vi "BuildInstaller.vi"(6 "VersionString":string, 8 "error in":errorcluster, 9 "DestinationDir":path, 10 "BuildSpec":string, 11 "ProjectPath":path=path "C:/Users/pauloneill/SCC/Orion/LabVIEW/Source/App/Orion.lvproj") -> (0 "error out":errorcluster, 3 "Generated files":path[](array[path]))   [LabVIEW 2020, in "CICD.lvlib"]
doc: "Build Windows Installer."
uses:
  CICD.lvlib
  <vilib>/AppBuilder/AB_API_Simple/NI_App_Builder_API.lvlib
  <vilib>/AppBuilder/AB_API_Simple/Build (path).vi
  <vilib>/AppBuilder/AB_API_Simple/Set Build Specification Version (path).vi
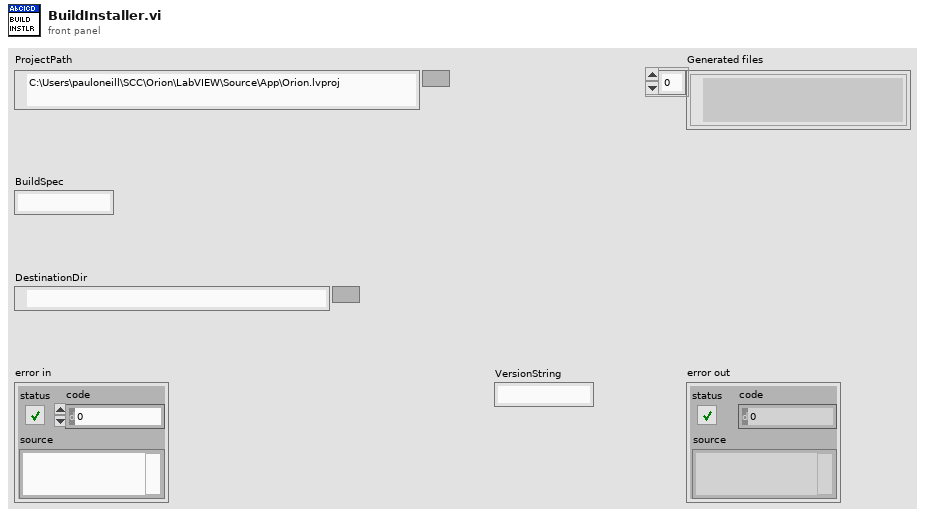
[diagram p1: front panel]
types:
  T1 = typedef "NI_App_Builder_API.lvlib/Build Specification Version.ctl" = cluster{"Major":u16, "Minor":u16, "Fix":u16, "Build":u16}
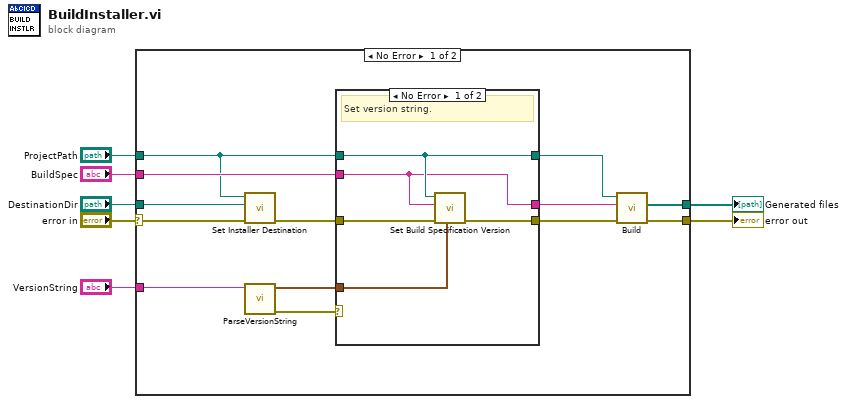
[diagram p0: block diagram]
diagram:
  n1 = case shown="No Error" "error in" {
    selector: "error in" -> [w12 w29]
    tunnel: [w19 w29] -> w7
    tunnel: "ProjectPath" -> [w10 _]
    tunnel: "BuildSpec" -> [w17 _]
    tunnel: "VersionString" -> [w16 _]
    tunnel: [w13 _] -> w3
    tunnel: "DestinationDir" -> [w9 _]
    frame No Error {
      n2 = call "Set Installer Destination.vi"("error in"=w12, "INST_buildLocation"=w9, ".lvproj"=w10) -> ("error out"=w11:errorcluster)  [unwired: 8 in]
      n3 = call "ParseVersionString.vi"("VersionString"=w16) -> ("error out"=w18:errorcluster, "Build spec version"=w8:T1)  [unwired: 9 in]
      n4 = case shown="No Error" w18 {
        tunnel: [w25 w28] -> w20
        tunnel: w11 -> [w21 w28]
        tunnel: w10 -> [w24 w27]
        tunnel: w17 -> [w23 w26]
        tunnel: [w24 w27] -> w15
        tunnel: [w23 w26] -> w14
        tunnel: w8 -> [w22 _]
        frame No Error {
          # "Set version string."
          n5 = call-poly <vilib>:"Set Build Specification Version.vi"("Build Specification Version"=w22, "error in (no error)"=w21, "Name of build specification"=w23, "Path to project"=w24) -> ("error out"=w25:errorcluster)  [unwired: 7 in]
        }
        frame Error {
          # "Could not parse version string."
        }
      }
      n6 = call-poly <vilib>:"Build.vi"("error in (no error)"=w20, "Name of build specification (if empty: build all)"=w14, "Path to project"=w15) -> ("error out"=w19:errorcluster, "Generated files"=w13:path[])  [unwired: 7 in]
    }
    frame Error {
    }
  }
  "error out" <- w7
  "Generated files" <- w3
